vi "EOL Calculate Vent AP data.vi"(8 "Truncation End":i32=15, 9 "Truncation Start":i32=15, 10 "Array Data":dbl[](array[numeric])) -> (3 "Vent Force calculated value":dbl)   [LabVIEW 2018]
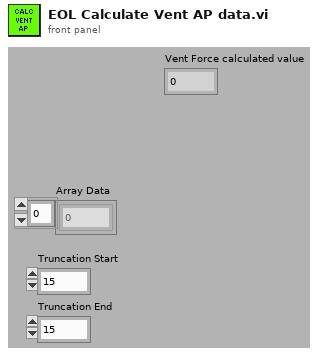
[diagram p1: front panel]
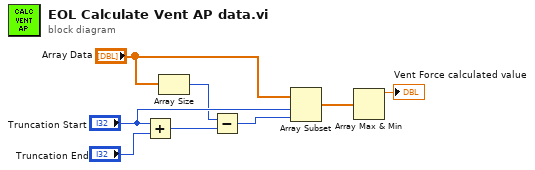
[diagram p0: block diagram]
diagram:
  n1 = Add(x="Truncation Start", y="Truncation End") -> (x+y=w5:i32)
  n2 = Array Size(array="Array Data") -> (size(s)=w6:i32)
  n3 = Subtract(x=w6, y=w5) -> (x-y=w4:i32)
  n4 = Array Subset(array="Array Data", index="Truncation Start", length=w4) -> (w2:dbl[])
  n5 = Array Max & Min(array=w2) -> (max value=→"Vent Force calculated value":dbl)  [unwired: 3 out]
